vi "TOP BOTTOM Timestamp.vi"(4 "Format":enum16{"at TOP", "at BOTTOM", "none"}(ring), 5 "Plot Bounds":T2, 6 "Timestamp":dbl, 7 "pixel center":cluster{"horizontal":i16, "vertical":i16}, 8 "time format (%H:%M:%S)":string="%I:%M:%S %p", 9 "GraphBGK":u32(colorbox), 10 "font":T1, 11 "new picture in":picture) -> (3 "new picture out":picture)   [LabVIEW 2018]
uses:
  <vilib>/Utility/miscctls.llb/LVRectTypeDef.ctl
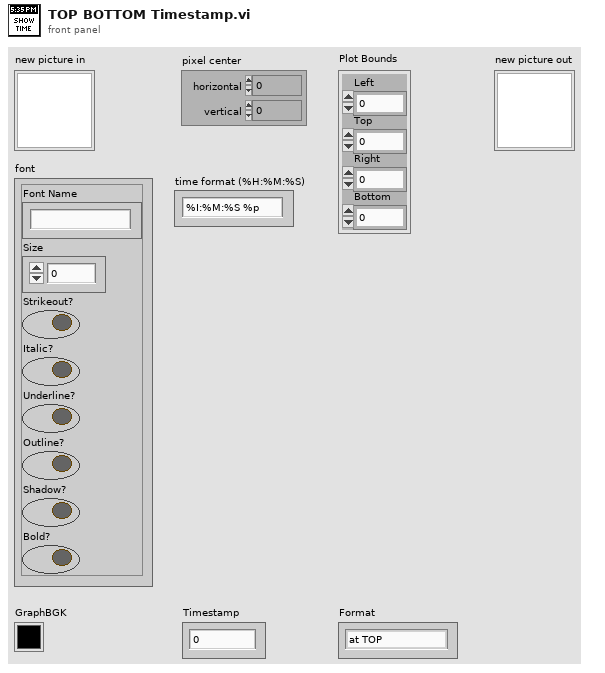
[diagram p1: front panel]
types:
  T1 = cluster{"Font Name":string, "Size":i16, "Strikeout?":bool, "Italic?":bool, "Underline?":bool, "Outline?":bool, "Shadow?":bool, "Bold?":bool}
  T2 = typedef "LVRectTypeDef.ctl" = cluster{"Left":i16, "Top":i16, "Right":i16, "Bottom":i16}
  T3 = enum16{"User-specified Font", "Application Font", "System Font", "Dialog Font"}
  T4 = cluster{"horizontal":enum16{"left", "center", "right"}, "vertical":enum16{"top", "center", "bottom"}}
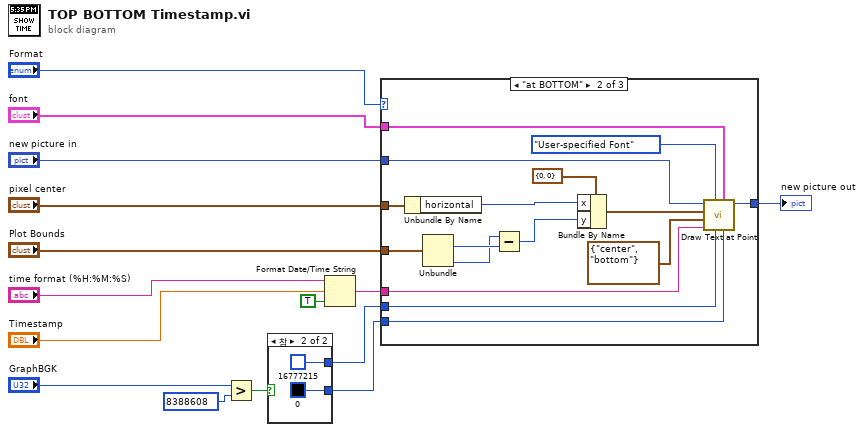
[diagram p0: block diagram]
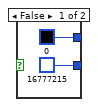
[diagram p2: hidden frame]
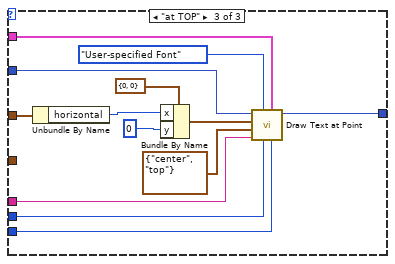
[diagram p4: hidden frame]
diagram:
  n1 = Greater?(x="GraphBGK", y=u32 8388608) -> (0:w10:bool)
  n2 = case shown="참" w10 {
    tunnel: [u32 0 u32 16777215] -> w7
    tunnel: [u32 16777215 u32 0] -> w6
    frame False {
    }
    frame True {
    }
  }
  n3 = Format Date/Time String(time format string (%c)="time format (%H:%M:%S)", seconds (now)="Timestamp", UTC format=TRUE ("세계시 포맷")) -> (date/time string=w2:string)
  n4 = case shown="\"at BOTTOM\"" "Format" {
    tunnel: w2 -> [_ w21 w37]
    tunnel: "Plot Bounds" -> [_ w30 _]
    tunnel: "pixel center" -> [_ w29 w49]
    tunnel: [w20 w35 w47] -> w12
    tunnel: "new picture in" -> [w20 w34 w46]
    tunnel: w7 -> [_ w25 w41]
    tunnel: w6 -> [_ w24 w40]
    tunnel: "font" -> [_ w22 w39]
    frame "none" {
    }
    frame "at BOTTOM" {
      n5 = Unbundle By Name(w29) -> ("horizontal"=w32:i16)
      n6 = Unbundle(w30) -> ("Top"=w28:i16, "Bottom"=w27:i16)  [unwired: 2 out]
      n7 = Subtract(x=w27, y=w28) -> (x-y=w26:i16)
      n8 = Bundle By Name(cluster=cluster{"x":i16, "y":i16} {"x"=0, "y"=0} ("origin"), "x"=w32, "y"=w26) -> (w33:cluster{"x":i16, "y":i16})
      n9 = call <vilib>:"Draw Text at Point.vi"("BG color(transparent)"=w24, "[user-specified font]"=w22, "text color(black)"=w25, "desired font(Application)"=T3."User-specified Font", "text"=w21, "alignment(left, top)"=T4 {"horizontal"=enum."center", "vertical"=enum."bottom"}, "origin"=w33, "picture"=w34) -> ("new picture"=w35:picture)  [unwired: 2 in, 1 out]
    }
    frame "at TOP" {
      n10 = Unbundle By Name(w49) -> ("horizontal"=w44:i16)
      n11 = Bundle By Name(cluster=cluster{"x":i16, "y":i16} {"x"=0, "y"=0} ("origin"), "x"=w44, "y"=i16 0) -> (w45:cluster{"x":i16, "y":i16})
      n12 = call <vilib>:"Draw Text at Point.vi"("BG color(transparent)"=w40, "[user-specified font]"=w39, "text color(black)"=w41, "desired font(Application)"=T3."User-specified Font", "text"=w37, "alignment(left, top)"=T4 {"horizontal"=enum."center", "vertical"=enum."top"}, "origin"=w45, "picture"=w46) -> ("new picture"=w47:picture)  [unwired: 2 in, 1 out]
    }
  }
  "new picture out" <- w12
